vi "AFPP Post-Uninstall Custom Action.vi"(10 "Variant":variant) -> (0 "error out":errorcluster)   [LabVIEW 2020]
uses:
  <vilib>/zip/NI_Unzip.lvlib
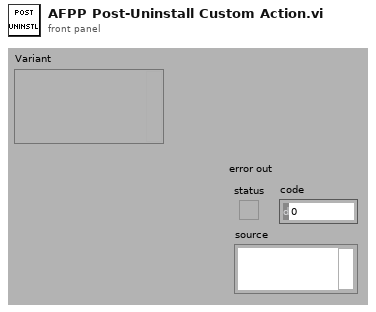
[diagram p1: front panel]
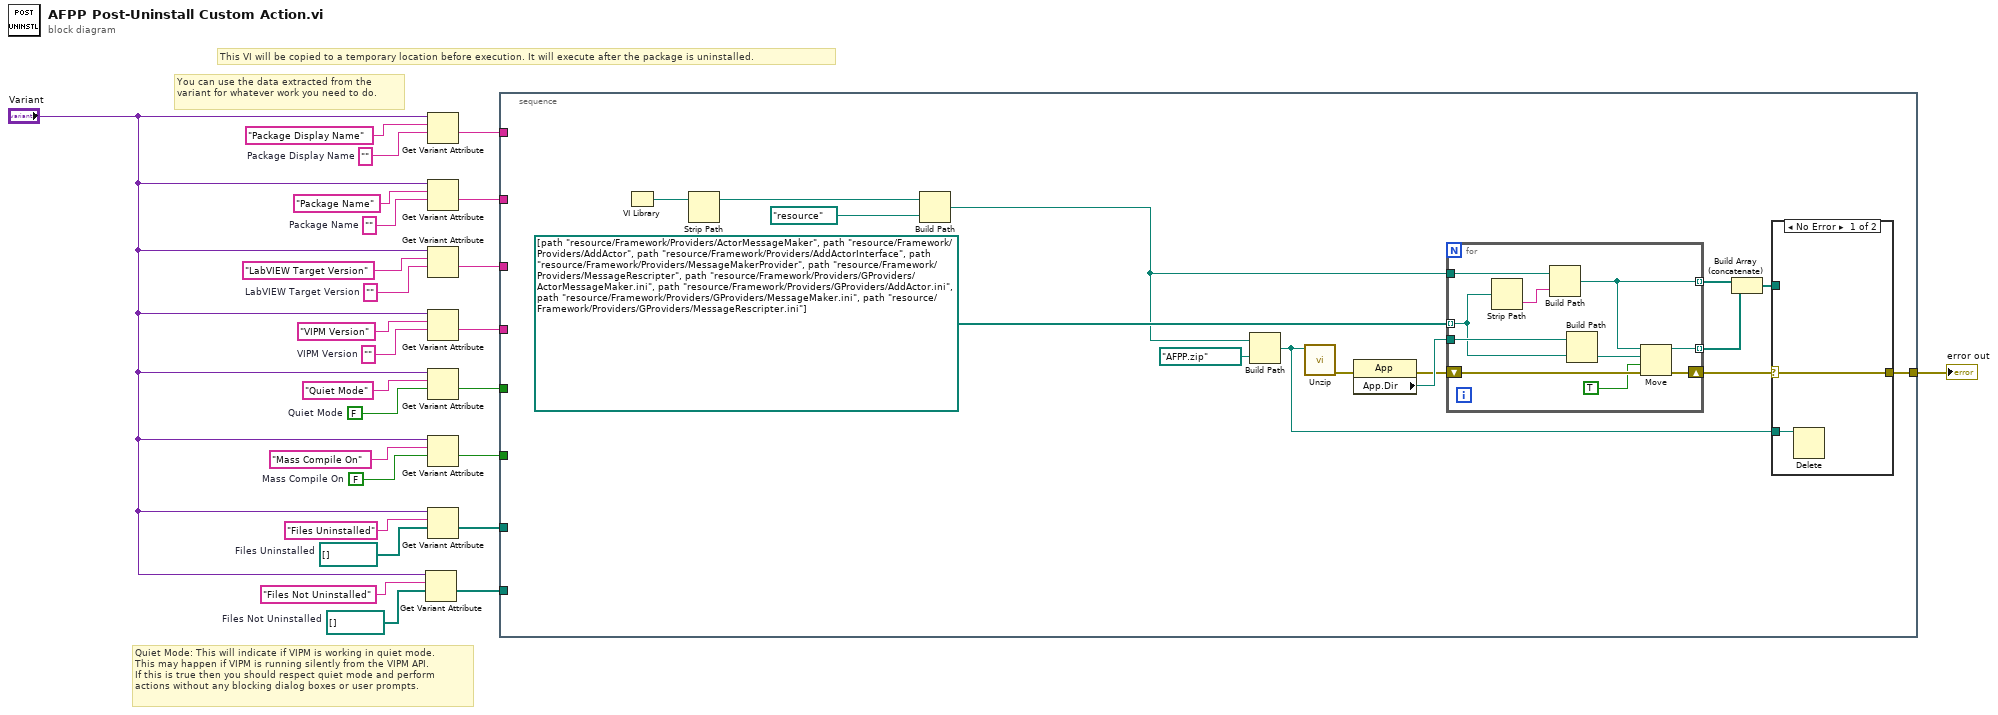
[diagram p0: block diagram]
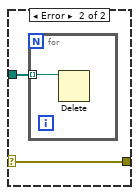
[diagram p2: hidden frame]
diagram:
  w2 = path[] []  # Files Not Uninstalled
  w3 = path[] []  # Files Uninstalled
  w9 = FALSE  # Mass Compile On
  w10 = ""  # Package Display Name
  w17 = FALSE  # Quiet Mode
  w20 = ""  # VIPM Version
  w22 = ""  # LabVIEW Target Version
  w24 = ""  # Package Name
  # "You can use the data extracted from the variant for whatever work you need to do."
  # "Quiet Mode: This will indicate if VIPM is working in quiet mode.\nThis may happen if VIPM is running silently from the VIPM API.\nIf this is true then you should respect quiet mode and perform\nactions without any blocking dialog boxes or user prompts."
  # "This VI will be copied to a temporary location before execution. It will execute after the package is uninstalled."
  n1 = Get Variant Attribute(Variant="Variant", name="Files Not Uninstalled", default value (empty Variant)=w2) -> (value=w7:path[])  [unwired: 1 in, 3 out]
  n2 = Get Variant Attribute(Variant="Variant", name="Package Display Name", default value (empty Variant)=w10) -> (value=w16:string)  [unwired: 1 in, 3 out]
  n3 = Get Variant Attribute(Variant="Variant", name="Package Name", default value (empty Variant)=w24) -> (value=w15:string)  [unwired: 1 in, 3 out]
  n4 = Get Variant Attribute(Variant="Variant", name="LabVIEW Target Version", default value (empty Variant)=w22) -> (value=w14:string)  [unwired: 1 in, 3 out]
  n5 = Get Variant Attribute(Variant="Variant", name="VIPM Version", default value (empty Variant)=w20) -> (value=w13:string)  [unwired: 1 in, 3 out]
  n6 = Get Variant Attribute(Variant="Variant", name="Quiet Mode", default value (empty Variant)=w17) -> (value=w12:bool)  [unwired: 1 in, 3 out]
  n7 = Get Variant Attribute(Variant="Variant", name="Mass Compile On", default value (empty Variant)=w9) -> (value=w11:bool)  [unwired: 1 in, 3 out]
  n8 = Get Variant Attribute(Variant="Variant", name="Files Uninstalled", default value (empty Variant)=w3) -> (value=w6:path[])  [unwired: 1 in, 3 out]
  n9 = stacked-sequence {
    tunnel: w16 -> [_]
    tunnel: w15 -> [_]
    tunnel: w14 -> [_]
    tunnel: w13 -> [_]
    tunnel: w12 -> [_]
    tunnel: w11 -> [_]
    tunnel: w6 -> [_]
    tunnel: w7 -> [_]
    tunnel: [w41] -> w1
    frame #0 {
      n10 = VI Library() -> (path=w30:path)
      n11 = Strip Path(path=w30) -> (stripped path=w28:path)  [unwired: 1 out]
      n12 = Build Path(base path=w28, name or relative path=path "resource") -> (appended path=w27:path)
      n13 = Build Path(base path=w27, name or relative path=path "AFPP.zip") -> (appended path=w40:path)
      n14 = call <vilib>:"Unzip.vi"("Zip file"=w40) -> ("error out"=w33:errorcluster)  [unwired: 8 in, 2 out]
      n15 = property class="App"(error in=w33) -> (error out=w34:errorcluster, "App.Dir"=w35:path)  [unwired: 1 in, 1 out]
      n16 = for {
        tunnel: w27 -> [w55]
        shift-right: [w54] -> w39
        shift-left: w34 -> [w56]
        tunnel: path[] [path "resource/Framework/Providers/ActorMessageMaker", path "resource/Framework/Providers/AddActor", path "resource/Framework/Providers/AddActorInterface", path "resource/Framework/Providers/MessageMakerProvider", path "resource/Framework/Providers/MessageRescripter", path "resource/Framework/Providers/GProviders/ActorMessageMaker.ini", path "resource/Framework/Providers/GProviders/AddActor.ini", path "resource/Framework/Providers/GProviders/MessageMaker.ini", path "resource/Framework/Providers/GProviders/MessageRescripter.ini"] -> [w51] mode=indexing
        tunnel: w35 -> [w52]
        tunnel: [w48] -> w36 mode=indexing
        tunnel: [w47] -> w38 mode=indexing
        n17 = Strip Path(path=w51) -> (name=w50:string)  [unwired: 1 out]
        n18 = Build Path(base path=w55, name or relative path=w50) -> (appended path=w48:path)
        n19 = Build Path(base path=w52, name or relative path=w51) -> (appended path=w53:path)
        n20 = Move(source path=w48, error in=w56, 9:TRUE ("overwrite (F)"), 10:w53) -> (error out=w54:errorcluster, 3:w47:path)  [unwired: 1 in, 1 out]
      }
      n21 = Build Array (concatenate)(w36, w38) -> (w37:path[])
      n22 = case shown="No Error" w39 {
        selector: w39 -> [w42 w44]
        tunnel: w37 -> [_ w45]
        tunnel: [w42 w44] -> w41
        tunnel: w40 -> [w43 _]
        frame No Error {
          n23 = Delete(path (use dialog)=w43) -> ()  [unwired: 4 in, 3 out]
        }
        frame Error {
          n24 = for {
            tunnel: w45 -> [w46] mode=indexing
            n25 = Delete(path (use dialog)=w46) -> ()  [unwired: 4 in, 3 out]
          }
        }
      }
    }
  }
  "error out" <- w1
